vi "MQTT_SubAck_Read.vi"(8 "error in (no error)":errorcluster, 11 "connection ID":refnum<k5>) -> (0 "error out":errorcluster, 1 "Granted QoS Levels":T1[](array[typedef]), 3 "connection ID out":refnum<k5>)   [LabVIEW 2017, in "MQTT_Functions.lvlib"]
doc: "© 2015 - daq.io, LLC - Peter Adelhardt"
uses:
  MQTT_Functions.lvlib
  Controls/QoS.ctl
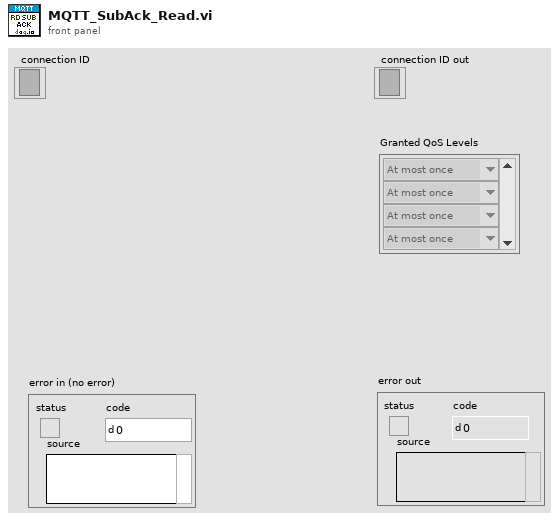
[diagram p1: front panel]
types:
  T1 = typedef "MQTT_Functions.lvlib/QoS.ctl" = enum8{"At most once", "At least once", "Exactly once", "Reserved"}
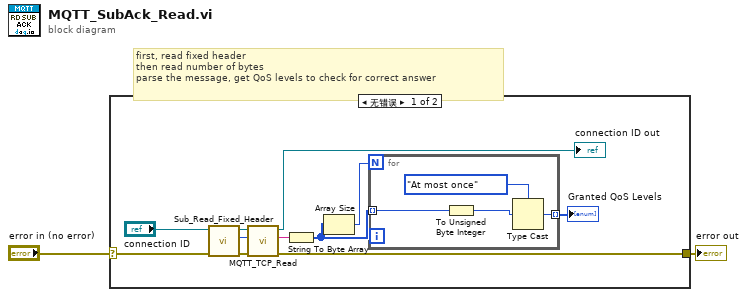
[diagram p0: block diagram]
diagram:
  # "first, read fixed header\nthen read number of bytes\nparse the message, get QoS levels to check for correct answer"
  n1 = case shown="无错误" "error in (no error)" {
    selector: "error in (no error)" -> [w6 w18]
    tunnel: [w4 w18] -> w1
    frame No Error {
      n2 = call "Sub_Read_Fixed_Header.vi"("error in (no error)"=w6, "connection ID"="connection ID") -> ("error out"=w5:errorcluster, "Remaining Length"=w9:u32, "connection ID out"=w8:refnum<k5>)  [unwired: 3 in, 4 out]
      n3 = call "MQTT_TCP_Read.vi"("error in (no error)"=w5, "bytes to read"=w9, "connection ID"=w8) -> ("error out"=w4:errorcluster, "data out"=w10:string, "connection ID out"=→"connection ID out":refnum<k5>)  [unwired: 6 in]
      n4 = String To Byte Array(string=w10) -> (unsigned byte array=w3:u8[])
      n5 = Array Size(array=w3) -> (size(s)=w12:i32)
      n6 = for {
        N: w12 -> [_]
        tunnel: [w16] -> w13 mode=indexing
        tunnel: w3 -> [w15] mode=indexing
        n7 = To Unsigned Byte Integer(number=w15) -> (unsigned 8bit integer=w14:u8)
        n8 = Type Cast(type=QoS."At most once" ("QoS Level"), x=w14) -> (*(type *) &x=w16:T1)
      }
      "Granted QoS Levels" <- w13
    }
    frame Error {
    }
  }
  "error out" <- w1
